vi "Main_SAIDD.vi"() -> ()   [LabVIEW 2018]
uses:
  <extravilib>/ChannelInstances/Tag-bool.lvlib
  <vilib>/myRIO/Instrument Drivers/Onboard IO/DIO/DIO.lvlib
  <vilib>/myRIO/Instrument Drivers/Onboard IO/PWM/PWM.lvlib
  <vilib>/myRIO/Instrument Drivers/Utilities/Utilities.lvlib
panel:
  out "Distance [cm]":dbl
  in  "Antal iterationer pr. stepper":i32=800
  in  "Stop":bool
  out "Measured current":dbl
  out "Ammeter measurement":dbl(graph)
  out "Duty Cycle":dbl
  out "Mean 200":dbl format="%0.2f"
  out "Battery left (%)":dbl
  in  "Drill - Frequency [Hz]":dbl=200.0
  in  "Stepper frekvens ned":dbl=120.0
  in  "Ingen modstand ned upper threshold":dbl=2750.0
  out "ALL TOP":bool
  out "ALL BOTTOM":bool
  in  "Resistance - Threshold Upper":dbl=3175.0
  in  "Resistance Threshold Lower":dbl=2975.0
  out "Process":T1(ring)
  in  "State":T1(ring)
  out "Image":T2(plugin-control)
  in  "high cutoff freq: fh":dbl=900.0
  in  "Radius":dbl=0.002 format="%#_13g"
  in  "Filter?":bool=TRUE
  out "RollDetection - Alarm":bool
  out "Data output (A3 GPS)":string[](array[string])
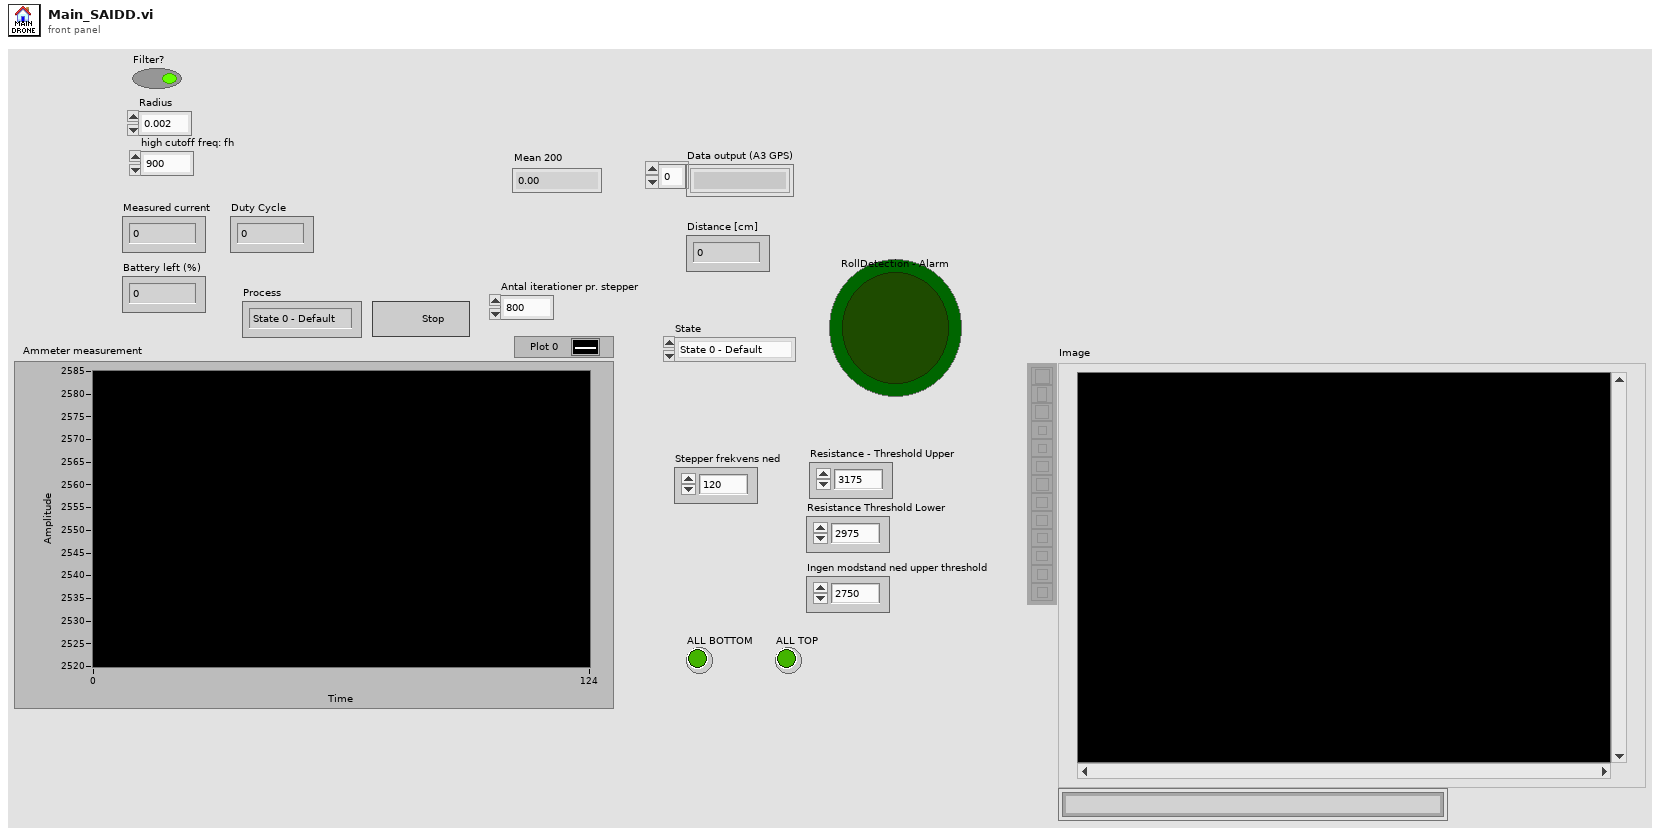
[diagram p1: front panel]
types:
  T1 = enum16{"State 0 - Default", "State 1 - Go down", "State 2 - Go up", "State 3 - Triangle Wobble"}
  T2 = typedef "IMAQ Image.ctl" = refnum<image>
  T3 = typedef "DIO.lvlib/DIO Reference.ctl" = cluster{"myRIO Reference":T4, "DIO Channels List":T8}
  T4 = typedef "myRIO Generic Hardware Reference.ctl" = cluster{"myRIO Model":T5, "myRIO Hardware Reference":T6}
  T5 = typedef "Hardware Version Enum.ctl" = enum16{"Unknown", "myRIO-1900", "myRIO-1950", "roboRIO", "NI ELVIS RIO CM", "ELVIS III"}
  T6 = typedef "myRIO v1.0 Reference.ctl" = cluster{"Generic FPGA Reference":T7, "Allow multiple opens":bool}
  T7 = typedef "Generic FPGA Reference.ctl" = refnum<k20>
  T8 = typedef "DIO Channels List.ctl" = T9[]
  T9 = typedef "DIO Channels Enum.ctl" = enum16{"Not Connected", "C/DIO0", "C/DIO1", "C/DIO2", "C/DIO3", "C/DIO4", "C/DIO5", "C/DIO6", "C/DIO7", "A/DIO0", "A/DIO1", "A/DIO2", "A/DIO3", "A/DIO4", "A/DIO5", "A/DIO6", "A/DIO7", "A/DIO8", "A/DIO9", "A/DIO10", "A/DIO11", "A/DIO12", "A/DIO13", "A/DIO14", "A/DIO15", "A/DIO16", "A/DIO17", "A/DIO18", "A/DIO19", "B/DIO0", "B/DIO1", "B/DIO2", "B/DIO3", "B/DIO4", "B/DIO5", "B/DIO6", "B/DIO7", "B/DIO8", "B/DIO9", "B/DIO10", "B/DIO11", "B/DIO12", "B/DIO13", "B/DIO14", "B/DIO15", "B/DIO16", "B/DIO17", "B/DIO18", "B/DIO19", "LED0", "LED1", "LED2", "LED3", "Button0", "DIO/DIO0", "DIO/DIO1", "DIO/DIO2", "DIO/DIO3", "DIO/DIO4", "DIO/DIO5", "DIO/DIO6", "DIO/DIO7", "DIO/DIO8", "DIO/DIO9", "SPI/CS0", "SPI/CS1", "SPI/CS2", "SPI/CS3", "LED RADIO (Green)", "LED RADIO (Red)", "LED COMM (Green)", "LED COMM (Red)", "LED MODE (Green)", "LED MODE (Red)"}
  T10 = typedef "PWM.lvlib/PWM Reference.ctl" = cluster{"myRIO Reference":T4, "PWM Channels Enum":T11, "PWM Configuration":T12}
  T11 = typedef "PWM Channels Enum.ctl" = enum16{"Not Connected", "C/PWM0", "C/PWM1", "A/PWM0", "A/PWM1", "A/PWM2", "A/PWM3", "A/PWM4", "A/PWM5", "A/PWM6", "A/PWM7", "A/PWM8", "A/PWM9", "A/PWM10", "A/PWM11", "A/PWM12", "A/PWM13", "A/PWM14", "A/PWM15", "A/PWM16", "A/PWM17", "A/PWM18", "A/PWM19", "B/PWM0", "B/PWM1", "B/PWM2", "B/PWM3", "B/PWM4", "B/PWM5", "B/PWM6", "B/PWM7", "B/PWM8", "B/PWM9", "B/PWM10", "B/PWM11", "B/PWM12", "B/PWM13", "B/PWM14", "B/PWM15", "B/PWM16", "B/PWM17", "B/PWM18", "B/PWM19", "PWM/PWM0", "PWM/PWM1", "PWM/PWM2", "PWM/PWM3", "PWM/PWM4", "PWM/PWM5", "PWM/PWM6", "PWM/PWM7", "PWM/PWM8", "PWM/PWM9"}
  T12 = typedef "PWM.lvlib/PWM Configuration.ctl" = cluster{"Frequency":dbl, "Duty Cycle":dbl}
  T13 = typedef "Accelerometer.lvlib/Accelerometer Reference.ctl" = cluster{"myRIO Reference":T4, "Accelerometer Channels List":T14, "LSB Weight":dbl}
  T14 = typedef "Accelerometer Channels List.ctl" = T15[]
  T15 = typedef "Accelerometer Channels Enum.ctl" = enum16{"Not Connected", "X-Axis", "Y-Axis", "Z-Axis"}
  T16 = typedef "AI.lvlib/AI Reference.ctl" = cluster{"myRIO Reference":T4, "AI Channels List":T17, "AI Scaling Constants List":T19}
  T17 = typedef "AI Channels List.ctl" = T18[]
  T18 = typedef "AI Channels Enum.ctl" = enum16{"Not Connected", "AudioIn/Left", "AudioIn/Right", "C/AI0", "C/AI1", "A/AI0", "A/AI1", "A/AI2", "A/AI3", "A/AI4", "A/AI5", "A/AI6", "A/AI7", "B/AI0", "B/AI1", "B/AI2", "B/AI3", "B/AI4", "B/AI5", "B/AI6", "B/AI7", "AI/AI0", "AI/AI1", "AI/AI2", "AI/AI3", "A/AI0 (DIFF)", "A/AI1 (DIFF)", "A/AI2 (DIFF)", "A/AI3 (DIFF)", "B/AI0 (DIFF)", "B/AI1 (DIFF)", "B/AI2 (DIFF)", "B/AI3 (DIFF)"}
  T19 = typedef "Analog Scaling Constants List.ctl" = T20[]
  T20 = typedef "Analog Scaling Constants.ctl" = cluster{"LSB Weight (Volts)":dbl, "Offset (Volts)":dbl, "Signed?":bool}
  T21 = typedef "SPI.lvlib/SPI Reference.ctl" = cluster{"myRIO Reference":T4, "SPI Channels Enum":T22, "SPI Configuration":T23}
  T22 = typedef "SPI Channels Enum.ctl" = enum16{"Not Connected", "A/SPI", "B/SPI", "SPI/SPI"}
  T23 = typedef "SPI.lvlib/SPI Configuration.ctl" = cluster{"Frequency [Hz]":dbl, "Clock Phase":T24, "Clock Polarity":T25, "Data Direction":T26, "Frame Length":T27}
  T24 = typedef "SPI Clock Phase.ctl" = enum8{"Leading", "Trailing"}
  T25 = typedef "SPI Clock Polarity.ctl" = enum8{"Low", "High"}
  T26 = typedef "SPI Data Direction.ctl" = enum8{"Most significant bit first", "Least significant bit first"}
  T27 = typedef "SPI Frame Length.ctl" = u8
  T28 = cluster{"B/DIO0 - Stepper Direction":T3, "B/DIO1 - Stepper1 Enable":T3, "B/DIO2 - Stepper2 Enable":T3, "B/DIO3 - Stepper3 Enable":T3, "B/DIO4 - Endstop Stepper1 Top":T3, "B/DIO11 - Endstop Stepper1 Bund":T3, "B/DIO12 - Endstop Stepper2 Top":T3, "B/DIO13 - Endstop Stepper2 Bund":T3, "B/DIO14 - Endstop Stepper3 Top":T3, "B/DIO15 - Endstop Stepper3 Bund":T3, "A/DIO0 - Cooler":T3, "A/DIO1 - Beacon drop (dio1)":T3, "A/DIO2 - Beacon drop (dio0)":T3, "A/DIO3 - QuickRelease (dio1)":T3, "A/DIO4 - QuickRelease (dio0)":T3, "A/DIO11 - LiDAR SPI CS":T3, "B/PWM0 - Stepper":T10, "B/PWM1 - Drill":T10, "A/PWM0 - Servo_Roll":T10, "A/PWM1 - Servo_Yaw":T10, "Acc. X-axis":T13, "Acc. Y-axis":T13, "B/AI0 - Drone Grounded S1 - F3":T16, "A/AI0 - QuickRelease S4 - F4":T16, "B/AI2 - Beacon Drop S5 - F5":T16, "B/AI3 - Begin drilling S3 - F6":T16, "B/AI1 - Gimbal Seach S8 - F8":T16, "A/AI1 - Beacon Wiper":T16, "A/AI2 - QuickRelease Wiper":T16, "A/AI3 - Drill Current":T16, "A/SPI - LiDAR":T21, "B/UART - XBee":refnum<visa-resource-name>, "A/UART - A3 GPS":refnum<visa-resource-name>, "RIO Flashing LEDs":T3}
  T29 = typedef "Tag-bool.lvlib/))Channel.ctl" = refnum<queue>
  T30 = typedef "IMAQdx.ctl" = refnum<k21>
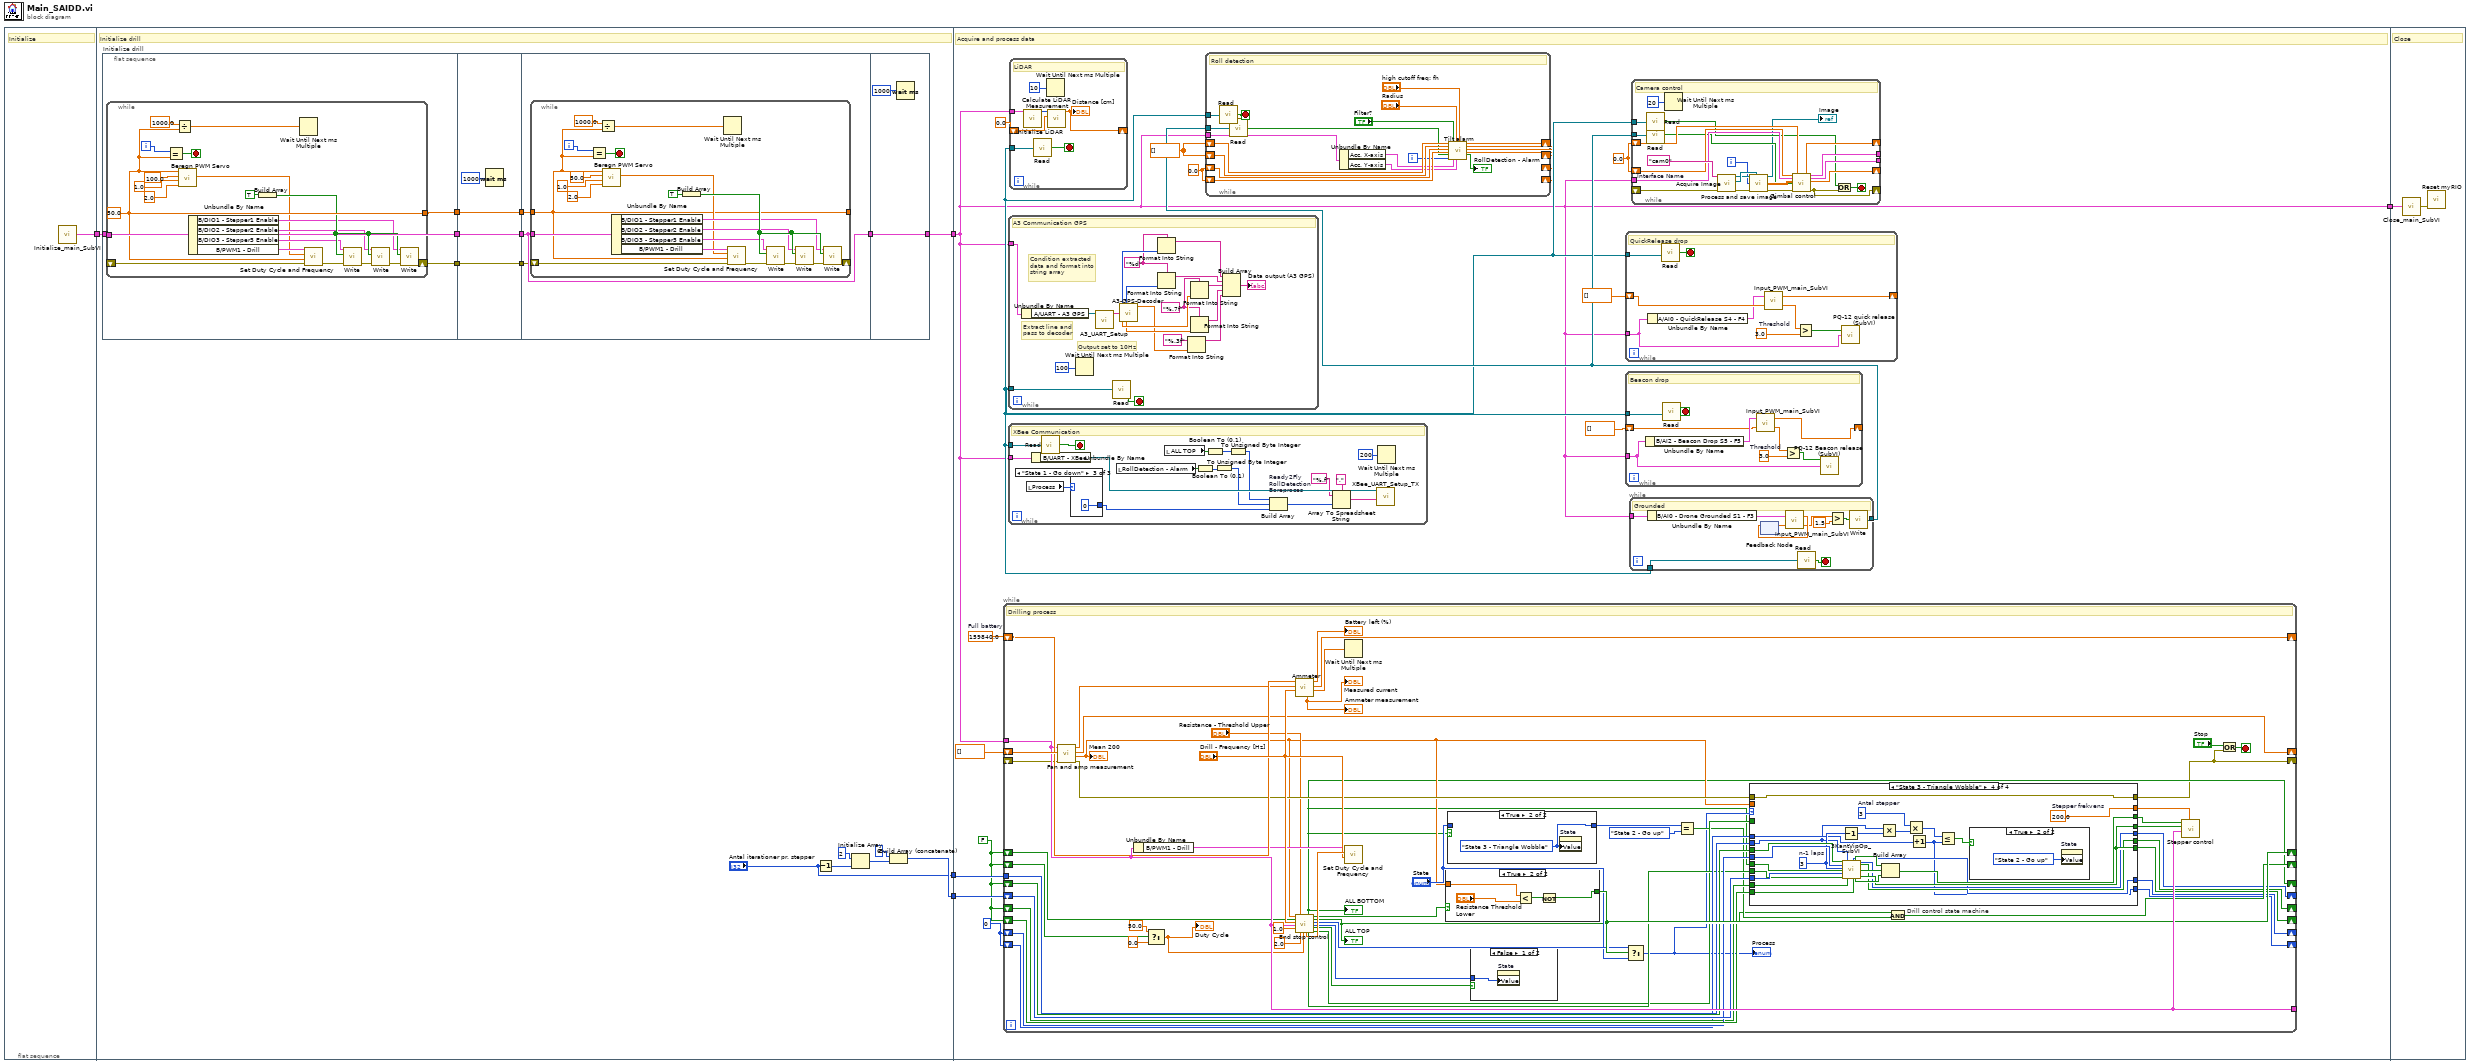
[diagram p0: block diagram]
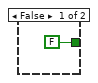
[diagram p4: hidden frame]
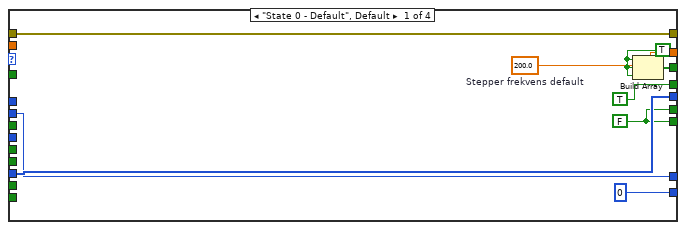
[diagram p5: hidden frame]
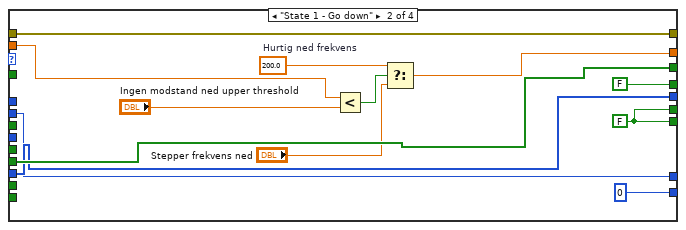
[diagram p6: hidden frame]
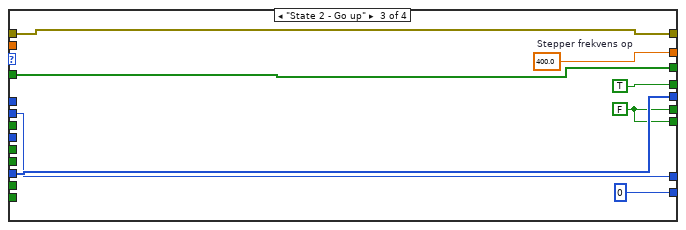
[diagram p7: hidden frame]
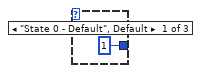
[diagram p9: hidden frame]
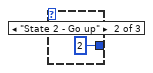
[diagram p10: hidden frame]
diagram:
  n1 = flat-sequence {
    tunnel: [w6] -> w4
    tunnel: w4 -> [w21]
    tunnel: [w18] -> w3
    tunnel: ["Antal iterationer pr. stepper"] -> w2
    tunnel: [w12] -> w1
    tunnel: w3 -> [w76]
    tunnel: [w76] -> w5
    tunnel: w2 -> [w82]
    tunnel: w1 -> [w81]
    tunnel: w5 -> [w331]
    frame #0 {
      # "Initialize"
      n2 = call "Initialize_main_SubVI.vi"() -> ("output cluster"=w6:T28)
    }
    frame #1 {
      # "Initialize drill"
      n3 = flat-sequence "Initialize drill" {
        tunnel: w21 -> [w24]
        tunnel: [w24] -> w20
        tunnel: [w23] -> w9
        tunnel: [w22] -> w7
        tunnel: w20 -> [w49]
        tunnel: [w49] -> w19
        tunnel: [w47] -> w10
        tunnel: w9 -> [w47]
        tunnel: [w46] -> w8
        tunnel: w7 -> [w46]
        tunnel: w19 -> [w52]
        tunnel: [w52] -> w17
        tunnel: w10 -> [w51]
        tunnel: w8 -> [w50]
        tunnel: [w75] -> w18
        tunnel: w17 -> [w75]
        frame #0 {
          n4 = while {
            tunnel: [w39] -> w23
            shift-right: [w31] -> w22
            shift-left: _ -> [w42]
            tunnel: w24 -> [w36]
            i -> [w41]
            stop <- w37 stop-if-true
            w39 = 50.0 ("Frequency [Hz]")
            n5 = Equal?(x=w41, y=w39) -> (x = y?=w37:bool)
            n6 = Divide(x=1000.0, y=w39) -> (x/y=w40:dbl)
            n7 = call "Beregn PWM Servo.vi"("Max (ms puls bredde)"=2.0, "Min (ms puls bredde)"=1.0, "Duty Cycle"=100.0, "Frekvens"=w39) -> ("Output Dutycycle til PWM Servo"=w25:dbl)  [unwired: 7 in]
            n8 = Unbundle By Name(w36) -> ("B/DIO1 - Stepper1 Enable"=w26:T3, "B/DIO2 - Stepper2 Enable"=w27:T3, "B/DIO3 - Stepper3 Enable"=w28:T3, "B/PWM1 - Drill"=w30:T10)
            n9 = Build Array(TRUE) -> (w29:bool[])
            n10 = Wait Until Next ms Multiple(millisecond multiple=w40) -> ()  [unwired: 1 out]
            n11 = call <vilib>:"Set Duty Cycle and Frequency.vi"("error in (no error)"=w42, "Frequency [Hz]"=w39, "Duty Cycle"=w25, "PWM Ref In"=w30) -> ("error out"=w34:errorcluster)  [unwired: 5 in, 1 out]
            n12 = call <vilib>:"Write.vi"("error in (no error)"=w34, "Values"=w29, "DIO Ref In"=w28) -> ("error out"=w33:errorcluster)  [unwired: 6 in, 1 out]
            n13 = call <vilib>:"Write.vi"("error in (no error)"=w33, "Values"=w29, "DIO Ref In"=w27) -> ("error out"=w32:errorcluster)  [unwired: 6 in, 1 out]
            n14 = call <vilib>:"Write.vi"("error in (no error)"=w32, "Values"=w29, "DIO Ref In"=w26) -> ("error out"=w31:errorcluster)  [unwired: 6 in, 1 out]
          }
        }
        frame #1 {
          n15 = Wait (ms)(milliseconds to wait=u32 1000) -> ()  [unwired: 1 out]
        }
        frame #2 {
          n16 = while {
            tunnel: [w53] -> _
            shift-right: [w60] -> _
            shift-left: w50 -> [w70]
            tunnel: w52 -> [w65]
            tunnel: w51 -> [w53]
            i -> [w69]
            stop <- w66 stop-if-true
            n17 = Equal?(x=w69, y=w53) -> (x = y?=w66:bool)
            n18 = Divide(x=1000.0, y=w53) -> (x/y=w68:dbl)
            n19 = call "Beregn PWM Servo.vi"("Max (ms puls bredde)"=2.0, "Min (ms puls bredde)"=1.0, "Duty Cycle"=50.0, "Frekvens"=w53) -> ("Output Dutycycle til PWM Servo"=w54:dbl)  [unwired: 7 in]
            n20 = Unbundle By Name(w65) -> ("B/DIO1 - Stepper1 Enable"=w55:T3, "B/DIO2 - Stepper2 Enable"=w56:T3, "B/DIO3 - Stepper3 Enable"=w57:T3, "B/PWM1 - Drill"=w59:T10)
            n21 = Build Array(TRUE) -> (w58:bool[])
            n22 = Wait Until Next ms Multiple(millisecond multiple=w68) -> ()  [unwired: 1 out]
            n23 = call <vilib>:"Set Duty Cycle and Frequency.vi"("error in (no error)"=w70, "Frequency [Hz]"=w53, "Duty Cycle"=w54, "PWM Ref In"=w59) -> ("error out"=w63:errorcluster)  [unwired: 5 in, 1 out]
            n24 = call <vilib>:"Write.vi"("error in (no error)"=w63, "Values"=w58, "DIO Ref In"=w57) -> ("error out"=w62:errorcluster)  [unwired: 6 in, 1 out]
            n25 = call <vilib>:"Write.vi"("error in (no error)"=w62, "Values"=w58, "DIO Ref In"=w56) -> ("error out"=w61:errorcluster)  [unwired: 6 in, 1 out]
            n26 = call <vilib>:"Write.vi"("error in (no error)"=w61, "Values"=w58, "DIO Ref In"=w55) -> ("error out"=w60:errorcluster)  [unwired: 6 in, 1 out]
          }
        }
        frame #3 {
          n27 = Wait (ms)(milliseconds to wait=u32 1000) -> ()  [unwired: 1 out]
        }
      }
      n28 = Decrement(x="Antal iterationer pr. stepper") -> (x-1=w16:i32)
      n29 = Initialize Array(2, w16) -> (w15:i32[])
      n30 = Build Array (concatenate)(6, w15) -> (w12:i32[])
    }
    frame #2 {
      w83 = 0.0 ("X-Stored-Shift-out")
      w84 = 0 ("Loops shift out")
      w80 = FALSE ("t")
      w86 = 159840.0  # Full battery
      w79 = 0.0 ("Position 2")
      w90 = dbl[] [] ("X-Array-Shift-out")
      # "Acquire and process data"
      n31 = while {
        shift-right: [w93] -> _
        shift-left: _ -> [w130]
        shift-right: [w98] -> _
        shift-left: dbl[] [] -> [w144]
        shift-right: [w140] -> _
        shift-left: w86 -> [w141]
        tunnel: w76 -> [w136]
        tunnel: [w136] -> _
        shift-right: [w132] -> _
        shift-left: w80 -> [w131]
        shift-right: [w128] -> _
        shift-left: w80 -> [w127]
        shift-right: [w125] -> _
        shift-left: w80 -> [w124]
        shift-right: [w123] -> _
        shift-left: w81 -> [w122]
        tunnel: w82 -> [w116]
        shift-right: [w120] -> _
        shift-left: w84 -> [w121]
        shift-right: [w119] -> _
        shift-left: w80 -> [w118]
        shift-right: [w95] -> _
        shift-left: w80 -> [w117]
        shift-right: [w114] -> _
        shift-left: w84 -> [w115]
        stop <- w92 stop-if-true
        # "Drilling process"
        n32 = call "Fan and amp measurement.vi"("error in (no error)"=w130, "Array in"=w144, "output cluster"=w136) -> ("error out"=w137:errorcluster, "Mean out"=w97:dbl, "Array out"=w98:dbl[], "dbl Scaled Value"=w134:dbl)  [unwired: 5 in]
        "Mean 200" <- w97
        n33 = Unbundle By Name(w136) -> ("B/PWM1 - Drill"=w138:T10)
        n34 = Select(t=50.0, s=w127, f=0.0 ("upper limit")) -> (s? t:f=w94:dbl)
        "Duty Cycle" <- w94
        n35 = call "Ammeter.vi"("Bor - Frequency [Hz]"="Drill - Frequency [Hz]", "Måling ammeter"=w134, "Sum batteri shift in"=w141) -> ("Wait ud"=w133:dbl, "Sum batteri shift ud"=w140:dbl, "Batteri tilbage (%)"=→"Battery left (%)":dbl, "Målt ampere"=→"Measured current" →"Ammeter measurement":dbl)  [unwired: 5 in]
        n36 = call "End stop control.vi"("Numeric"=w97, "t"=w131, "Bor - Frequency [Hz]"="Drill - Frequency [Hz]", "output cluster"=w136, "Min (ms puls bredde)"=1.0, "Threshold Upper"="Resistance - Threshold Upper", "Max (ms puls bredde)"=2.0, "Bor - Duty Cycle"=w94) -> ("Output Dutycycle til PWM Servo"=w143:dbl, "ALL BOTTOM"=w95:bool, "Array 2"=w111:bool[], "Boolean 3"=w108:bool, "ALL TOP"=w96:bool, "Enum 2"=w104:T1, "Enum"=w101:T1, "Boolean"=w102:bool, "Array"=w110:bool[])  [unwired: 3 in]
        "ALL TOP" <- w96
        "ALL BOTTOM" <- w95
        n37 = Wait Until Next ms Multiple(millisecond multiple=w133) -> ()  [unwired: 1 out]
        n38 = call <vilib>:"Set Duty Cycle and Frequency.vi"("Frequency [Hz]"="Drill - Frequency [Hz]", "Duty Cycle"=w143, "PWM Ref In"=w138) -> ()  [unwired: 6 in, 2 out]
        n39 = case shown="True" w108 {
          tunnel: [FALSE w151] -> w132
          tunnel: w97 -> [_ w153]
          frame False {
          }
          frame True {
            n40 = Less?(x=w153, y="Resistance Threshold Lower") -> (x < y?=w152:bool)
            n41 = Not(x=w152) -> (.not. x?=w151:bool)
          }
        }
        n42 = case shown="True" w95 {
          tunnel: [w148 w149] -> w107
          tunnel: "State" -> [w148 _]
          frame False {
          }
          frame True {
            w149 = T1."State 3 - Triangle Wobble" ("Enum")
            n43 = property on="State" class="Enum (strict)"("Value"=w149) -> ()  [unwired: 2 in, 2 out]
          }
        }
        n44 = case shown="False" w102 {
          tunnel: w101 -> [w147 _]
          frame False {
            n45 = property on="State" class="Enum (strict)"("Value"=w147) -> ()  [unwired: 2 in, 2 out]
          }
          frame True {
          }
        }
        n46 = Select(t=w104, s=w132, f="State") -> (s? t:f=w100:T1)
        "Process" <- w100
        n47 = Equal?(x=w107, y=T1."State 2 - Go up" ("Enum")) -> (x = y?=w106:bool)
        n48 = case "Drill control state machine" shown="\"State 3 - Triangle Wobble\"" w100 {
          tunnel: [w161 w176 w184 w205] -> w99
          tunnel: w111 -> [_ w176 _ w196]
          tunnel: w110 -> [_ _ w184 _]
          tunnel: [TRUE FALSE TRUE w204] -> w135
          tunnel: w137 -> [w160 w174 w182 w209]
          tunnel: [w160 w174 w182 w209] -> w93
          tunnel: [w159 w171 w181 w210] -> w129
          tunnel: w97 -> [_ w168 _ _]
          tunnel: [w156 w165 w178 w204] -> w125
          tunnel: w124 -> [_ _ _ w203]
          tunnel: [w158 w167 w180 w202] -> w123
          tunnel: w122 -> [w158 w167 w180 w201]
          tunnel: w116 -> [w157 w166 w179 w190]
          tunnel: w121 -> [_ _ _ w200]
          tunnel: [w157 w166 w179 w199] -> w120
          tunnel: [w156 w165 w178 w198] -> w119
          tunnel: w118 -> [_ _ _ w197]
          tunnel: w117 -> [_ _ _ w195]
          tunnel: w95 -> [_ _ _ w193]
          tunnel: w115 -> [_ _ _ w192]
          tunnel: [0 0 0 w186] -> w114
          frame "State 0 - Default", Default {
            w156 = FALSE
            w159 = 200.0  # Stepper frekvens default
            w162 = TRUE
            n49 = Build Array(w162, w162, w162) -> (w161:bool[])
          }
          frame "State 1 - Go down" {
            w165 = FALSE
            w170 = 200.0  # Hurtig ned frekvens
            n50 = Less?(x=w168, y="Ingen modstand ned upper threshold") -> (x < y?=w173:bool)
            n51 = Select(t=w170, s=w173, f="Stepper frekvens ned") -> (s? t:f=w171:dbl)
          }
          frame "State 2 - Go up" {
            w178 = FALSE
            w181 = 400.0  # Stepper frekvens op
          }
          frame "State 3 - Triangle Wobble" {
            w188 = 3  # Antal stepper
            w194 = 3  # n-1 laps
            w210 = 200.0  # Stepper frekvens
            n52 = Decrement(x=w194) -> (x-1=w191:i32)
            n53 = call "3KantVipOp_SubVI.vi"("Shift 1 in"=w195, "Loops shift in"=w200, "n-1 omgange"=w194, "BUND!"=w193, "Index step array shift in"=w201, "Enable array"=w196, "Antal iterationer pr. stepper"=w190, "Shift 2 in"=w197, "Direction shift in"=w203) -> ("Loops shift out"=w199:i32, "Enable 1"=w206:bool, "Enable 3"=w208:bool, "Index step array shift ud"=w202:i32[], "Shift 2 ud"=w198:bool, "Enable 2"=w207:bool, "Direction shift ud"=w204:bool)  [unwired: 3 in, 1 out]
            n54 = Multiply(x=w190, y=w191) -> (x*y=w189:i32)
            n55 = Build Array(w206, w207, w208) -> (w205:bool[])
            n56 = Multiply(x=w188, y=w189) -> (x*y=w187:i32)
            n57 = Increment(x=w192) -> (x+1=w186:i32)
            n58 = Less Or Equal?(x=w187, y=w186) -> (x <= y?=w185:bool)
            n59 = case shown="True" w185 {
              frame False {
              }
              frame True {
                n60 = property on="State" class="Enum (strict)"("Value"=T1."State 2 - Go up" ("Enum")) -> ()  [unwired: 2 in, 2 out]
              }
            }
          }
        }
        n61 = And(x=w96, y=w106) -> (x .and. y?=w128:bool)
        n62 = call "Stepper control.vi"("Stepper frekvens"=w129, "output cluster"=w136, "Direction shift ud"=w135, "Array"=w99) -> ()  [unwired: 8 in]
        n63 = Or(x="Stop", y=w93) -> (x .or. y?=w92:bool)
      }
      n64 = while {
        tunnel: w76 -> [w252]
        tunnel: [w253] -> w78
        stop <- w254 stop-if-true
        w240 = "%.7f" ("format string")
        w241 = "%d" ("format string")
        # "Output set to 10Hz"
        # "Condition extracted\ndata and format into \nstring array"
        # "Extract line and\npass to decoder"
        # "A3 Communication GPS"
        n65 = Unbundle By Name(w252) -> ("A/UART - A3 GPS"=w236:refnum<visa-resource-name>)
        n66 = Wait Until Next ms Multiple(millisecond multiple=u32 100 ("milliseconds to wait")) -> ()  [unwired: 1 out]
        n67 = call "A3_UART_Setup.vi"("VISA Refnum in"=w236) -> ("read buffer"=w237:string)  [unwired: 9 in, 1 out]
        n68 = call <extravilib>:"Read.vi"("channel"=w253) -> ("element"=w254:bool)  [unwired: 1 in, 1 out]
        n69 = call "A3-GPS-Decoder.vi"("ASCII Hexidecimal String"=w237) -> ("Date (YYYYMMDD)"=w246:u32, "Time (HHMMSS)"=w245:u32, "Longitude (Deg)"=w244:dbl, "Latitude (Deg)"=w243:dbl, "AMSL (m)"=w242:sgl)  [unwired: 3 out]
        n70 = Format Into String(format string=w241, w246) -> (resulting string=w247:string)  [unwired: 2 in, 1 out]
        n71 = Format Into String(format string=w241, w245) -> (resulting string=w251:string)  [unwired: 2 in, 1 out]
        n72 = Format Into String(format string="%.3f", w242) -> (resulting string=w248:string)  [unwired: 2 in, 1 out]
        n73 = Format Into String(format string=w240, w244) -> (resulting string=w250:string)  [unwired: 2 in, 1 out]
        n74 = Format Into String(format string=w240, w243) -> (resulting string=w249:string)  [unwired: 2 in, 1 out]
        n75 = Build Array(w247, w251, w250, w249, w248) -> (→"Data output (A3 GPS)":string[])
      }
      n76 = while {
        tunnel: w78 -> [w270]
        tunnel: w76 -> [w269]
        stop <- w271 stop-if-true
        # "XBee Communication"
        n77 = local read "Process"() -> (w262:T1)
        n78 = Unbundle By Name(w269) -> ("B/UART - XBee"=w268:refnum<visa-resource-name>)
        n79 = call <extravilib>:"Read.vi"("channel"=w270) -> ("element"=w271:bool)  [unwired: 1 in, 1 out]
        n80 = case shown="\"State 1 - Go down\"" w262 {
          tunnel: [u8 1 u8 2 u8 0] -> w261
          frame "State 0 - Default", Default {
          }
          frame "State 2 - Go up" {
          }
          frame "State 1 - Go down" {
          }
        }
        n81 = local read "RollDetection - Alarm"() -> (w257:bool)
        n82 = local read "ALL TOP"() -> (w260:bool)
        n83 = Boolean To (0,1)(Boolean=w257) -> (0, 1=w256:i16)
        n84 = Boolean To (0,1)(Boolean=w260) -> (0, 1=w259:i16)
        n85 = To Unsigned Byte Integer(number=w256) -> (unsigned 8bit integer=w255:u8)
        n86 = To Unsigned Byte Integer(number=w259) -> (unsigned 8bit integer=w258:u8)
        n87 = Build Array "Ready2Fly\nRollDetection\nBoreproces"(w258, w255, w261) -> (w264:u8[])
        n88 = Array To Spreadsheet String(delimiter (Tab)=",", array=w264, 3:"%.f" ("format string")) -> (spreadsheet string=w267:string)
        n89 = call "XBee_UART_Setup_TX.vi"("Characters to Write"=w267, "VISA resource name in"=w268) -> ()  [unwired: 9 in, 1 out]
        n90 = Wait Until Next ms Multiple(millisecond multiple=u32 200) -> ()  [unwired: 1 out]
      }
      n91 = while {
        tunnel: w78 -> [w327]
        shift-right: [w325] -> _
        shift-left: 0.0 -> [w324]
        tunnel: w76 -> [w323]
        stop <- w326 stop-if-true
        # "LiDAR"
        n92 = call "Initialize LiDAR.vi"("output cluster"=w323) -> ("unsigned byte array"=w328:u8[])  [unwired: 10 in]
        n93 = call <extravilib>:"Read.vi"("channel"=w327) -> ("element"=w326:bool)  [unwired: 1 in, 1 out]
        n94 = Wait Until Next ms Multiple(millisecond multiple=u32 10) -> ()  [unwired: 1 out]
        n95 = call "Calculate LiDAR Measurement.vi"("Old distance"=w324, "unsigned byte array"=w328) -> ("New distance"=w325:dbl)  [unwired: 9 in]
        "Distance [cm]" <- w325
      }
      n96 = while {
        tunnel: w78 -> [w302]
        shift-right: [w301] -> _
        shift-left: dbl[] [] ("Shift out") -> [w300]
        tunnel: w76 -> [w296]
        stop <- w303 stop-if-true
        w299 = 3.0  # Threshold
        # "QuickRelease drop"
        n97 = Unbundle By Name(w296) -> ("A/AI0 - QuickRelease S4 - F4"=w297:T16)
        n98 = call <extravilib>:"Read.vi"("channel"=w302) -> ("element"=w303:bool)  [unwired: 1 in, 1 out]
        n99 = call "Input_PWM_main_SubVI.vi"("Shift in"=w300, "AI Ref In"=w297) -> ("Value out"=w298:dbl, "Shift out"=w301:dbl[])
        n100 = Greater?(x=w298, y=w299) -> (0:w295:bool)
        n101 = call "PQ-12 quick release (SubVI).vi"("output cluster"=w296, "Extend / Retract [F/T]"=w295) -> ()  [unwired: 1 in, 1 out]
      }
      n102 = while {
        tunnel: w76 -> [w315]
        tunnel: w78 -> [w321]
        shift-right: [w319] -> _
        shift-left: dbl[] [] ("Shift out") -> [w318]
        stop <- w322 stop-if-true
        w317 = 3.0  # Threshold
        # "Beacon drop"
        n103 = Unbundle By Name(w315) -> ("B/AI2 - Beacon Drop S5 - F5"=w320:T16)
        n104 = call <extravilib>:"Read.vi"("channel"=w321) -> ("element"=w322:bool)  [unwired: 1 in, 1 out]
        n105 = call "Input_PWM_main_SubVI.vi"("Shift in"=w318, "AI Ref In"=w320) -> ("Value out"=w316:dbl, "Shift out"=w319:dbl[])
        n106 = Greater?(x=w316, y=w317) -> (0:w314:bool)
        n107 = call "PQ-12 Beacon release (SubVI).vi"("output cluster"=w315, "Extend / Retract [T/F]"=w314) -> ()  [unwired: 1 in, 1 out]
      }
      n108 = while {
        tunnel: w78 -> [w312]
        tunnel: w76 -> [w311]
        tunnel: [w310] -> w87
        stop <- w313 stop-if-true
        # "Grounded"
        n109 = Unbundle By Name(w311) -> ("B/AI0 - Drone Grounded S1 - F3"=w305:T16)
        n110 = feedback #1() -> (w307:dbl[])  [unwired: 1 in]
        n111 = call "Input_PWM_main_SubVI.vi"("Shift in"=w307, "AI Ref In"=w305) -> ("Value out"=w306:dbl, "Shift out"=w308:dbl[])
        n112 = feedback-in #1(w308) -> ()
        n113 = call <extravilib>:"Read.vi"("channel"=w312) -> ("element"=w313:bool)  [unwired: 1 in, 1 out]
        n114 = Greater?(x=w306, y=1.5 ("x")) -> (0:w304:bool)
        n115 = call <vilib>:"Write.vi"("element"=w304) -> ("channel"=w310:T29)  [unwired: 1 out]
      }
      n116 = while {
        shift-right: [w289] -> _
        shift-left: w90 -> [w294]
        shift-right: [w288] -> _
        shift-left: w90 -> [w293]
        shift-right: [w287] -> _
        shift-left: w83 -> [w292]
        shift-right: [w286] -> _
        shift-left: w83 -> [w291]
        tunnel: w78 -> [w284]
        tunnel: w87 -> [w282]
        tunnel: w76 -> [w275]
        i -> [w290]
        stop <- w283 stop-if-true
        # "Roll detection"
        n117 = call <extravilib>:"Read.vi"("channel"=w284) -> ("element"=w283:bool)  [unwired: 1 in, 1 out]
        n118 = call <extravilib>:"Read.vi"("channel"=w282) -> ("element"=w281:bool)  [unwired: 1 in, 1 out]
        n119 = Unbundle By Name(w275) -> ("Acc. X-axis"=w279:T13, "Acc. Y-axis"=w280:T13)
        n120 = call "Tilt alarm.vi"("X-Array-Shift-in"=w294, "Y-Array-Shift-in"=w293, "X-Stored-Shift-in"=w292, "Y-Stored-Shift-in"=w291, "Grounded?"=w281, "Iterations"=w290, "Filter?"="Filter?", "Accelerometer Ref X in"=w279, "Radius"="Radius", "Accelerometer Ref Y In"=w280, "high cutoff freq: fh"="high cutoff freq: fh") -> ("X-Array-Shift-out"=w289:dbl[], "Y-Array-Shift-out"=w288:dbl[], "X-Stored-Shift-out"=w287:dbl, "Y-Stored-Shift-out"=w286:dbl, "Alarm"=→"RollDetection - Alarm":bool)  [unwired: 4 in]
      }
      n121 = while {
        shift-right: [w225] -> _
        shift-left: w79 -> [w226]
        shift-right: [w227] -> _
        shift-left: w79 -> [w228]
        tunnel: w76 -> [w219]
        tunnel: [w221] -> _
        tunnel: [w220] -> _
        tunnel: w78 -> [w218]
        tunnel: w87 -> [w215]
        shift-right: [w217] -> _
        shift-left: _ -> [w229]
        i -> [w224]
        stop <- w234 stop-if-true
        w232 = "cam0"  # Interface Name
        # "Camera control"
        n122 = call <extravilib>:"Read.vi"("channel"=w218) -> ("element"=w216:bool)  [unwired: 1 in, 1 out]
        n123 = call <extravilib>:"Read.vi"("channel"=w215) -> ("element"=w214:bool)  [unwired: 1 in, 1 out]
        n124 = Wait Until Next ms Multiple(millisecond multiple=u32 20 ("milliseconds to wait")) -> ()  [unwired: 1 out]
        n125 = call "Acquire Image.vi"("error in (no error)"=w229, "Interface Name"=w232) -> ("error out"=w233:errorcluster, "New Image"=w231:T2, "Refnum out"=w230:T30)  [unwired: 7 in]
        n126 = call "Process and save image.vi"("Refnum in"=w230, "New Image"=w231, "Numeric"=w224, "error in (no error)"=w233) -> ("Refnum out"=→"Image":T2, "Particle Measurements (Pixels)"=w222:dbl[][], "error out"=w223:errorcluster)  [unwired: 8 in, 1 out]
        n127 = call "Gimbal control.vi"("Position 5"=w228, "output cluster"=w219, "Particle Measurements (Pixels)"=w222, "element"=w214, "error in (no error)"=w223, "Position 3"=w226) -> ("Position 2"=w225:dbl, "PWM Ref Out 2"=w221:T10, "PWM Ref Out"=w220:T10, "Position 4"=w227:dbl, "error out"=w217:errorcluster)  [unwired: 6 in, 3 out]
        n128 = Or(x=w216, y=w217) -> (x .or. y?=w234:bool)
      }
    }
    frame #3 {
      # "Close"
      n129 = call "Close_main_SubVI.vi"("output cluster"=w331) -> ("error constant"=w330:errorcluster)
      n130 = call <vilib>:"Reset myRIO.vi"("error in (no error)"=w330) -> ()  [unwired: 10 in, 1 out]
    }
  }
